vi "FdxCountServerResourcesCvi.vi"(8 "error in":errorcluster, 11 "SrvName (local)":string="local") -> (0 "error out":errorcluster, 3 "Number of Resources":u32)   [LabVIEW 2020, in "AIM664LV.lvlib"]
doc: "This function is to get the number of AFDX boards of one computer or server."
uses:
  AIM664LV.lvlib
  FdxGlobalDllPath.vi
panel:
  out "Server Name Out":string
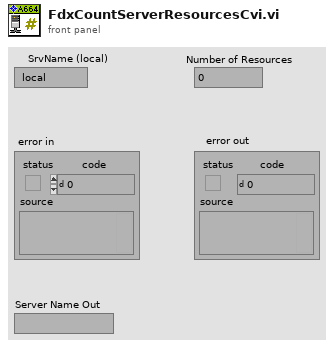
[diagram p1: front panel]
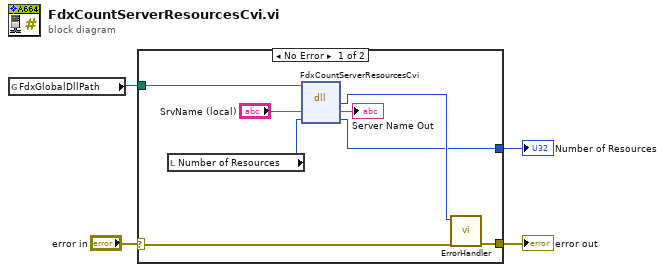
[diagram p0: block diagram]
diagram:
  n1 = global read "FdxGlobalDllPath.vi" "FdxGlobalDllPath"() -> (w2:path)
  n2 = case shown="No Error" "error in" {
    selector: "error in" -> [w11 w13]
    tunnel: [w12 w13] -> w4
    tunnel: w2 -> [w7 _]
    tunnel: [w6 _] -> w1
    frame No Error {
      n3 = local read "Number of Resources"() -> (w9:u32)
      n4 = dll-call lib="aim_fdx.19.dll" fn="FdxCountServerResourcesCvi"(path in=w7, "SrvName"="SrvName (local)", "NuOfResources"=w9) -> ("status"=w10:i32, "SrvName"=→"Server Name Out":string, "NuOfResources"=w6:u32)  [unwired: 2 in, 2 out]
      n5 = call "ErrorHandler.vi"("error in"=w11, "AIM Error"=w10) -> ("error out"=w12:errorcluster)  [unwired: 9 in]
    }
    frame Error {
    }
  }
  "error out" <- w4
  "Number of Resources" <- w1
